vi "KE_scan_create_cluster_for_graph.vi"(5 "Channel":i32=1 min=0 max=7 step=1, 7 "new data point":dbl[](array[numeric]), 8 "NI DAQ (t) / Keithley (f)":bool, 9 "iteration":i32, 10 "div I zero":bool=TRUE, 11 "KE scan in":dbl[][](array[numeric])) -> (2 "XY Graph Array":cluster{dbl[], "subarray":dbl[]}[](array[cluster]), 3 "KE scan out":dbl[][](array[numeric]))   [LabVIEW 2018]
panel:
  # "divide by other Keithley Channel"
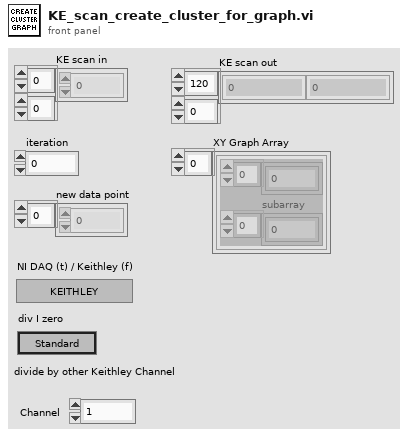
[diagram p1: front panel]
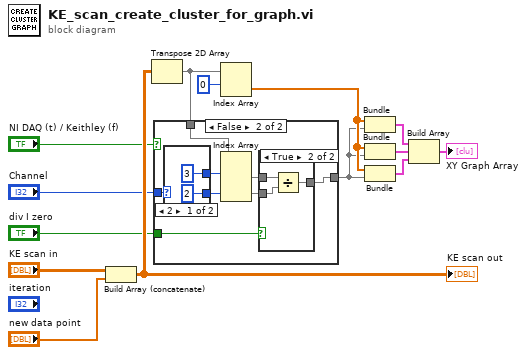
[diagram p0: block diagram]
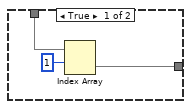
[diagram p2: hidden frame]
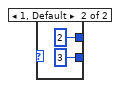
[diagram p3: hidden frame]
diagram:
  n1 = Build Array (concatenate)("KE scan in", "new data point") -> (w4:dbl[][])
  "KE scan out" <- w4
  n2 = Transpose 2D Array(2D array=w4) -> (transposed array=w13:dbl[][])
  n3 = case shown="False" "NI DAQ (t) / Keithley (f)" {
    tunnel: w13 -> [w16 w24]
    tunnel: [w15 w19] -> w7
    tunnel: "div I zero" -> [_ w20]
    tunnel: "Channel" -> [_ w18]
    frame True {
      n4 = Index Array(array=w16, index (row)=1) -> (element=w15:dbl[])  [unwired: 1 in]
    }
    frame False {
      n5 = case shown="2" w18 {
        tunnel: [3 ("index (row)") 2 ("index (row)")] -> w25
        tunnel: [2 ("index (row)") 3 ("index (row)")] -> w23
        frame 2 {
        }
        frame 1, Default {
        }
      }
      n6 = Index Array(array=w24, index (row) #1=w25, index (row) #2=w23) -> (element #1=w22:dbl[], element #2=w21:dbl[])  [unwired: 2 in]
      n7 = case shown="True" w20 {
        tunnel: w22 -> [w30 w33]
        tunnel: w21 -> [_ w32]
        tunnel: [w30 w31] -> w19
        frame False {
        }
        frame True {
          n8 = Divide(x=w33, y=w32) -> (x/y=w31:dbl[])
        }
      }
    }
  }
  n9 = Index Array(array=w13, index (row)=0) -> (element=w12:dbl[])  [unwired: 1 in]
  n10 = Bundle(w12, w7) -> (w11:cluster{dbl[], dbl[]})  [unwired: 1 in]
  n11 = Bundle(w12, w7) -> (w10:cluster{dbl[], dbl[]})  [unwired: 1 in]
  n12 = Bundle(w12, w7) -> (w9:cluster{dbl[], dbl[]})  [unwired: 1 in]
  n13 = Build Array(w11, w10, w9) -> (→"XY Graph Array":cluster{dbl[], dbl[]}[])
